vi "Actor Core.vi"(8 "error in":errorcluster, 11 "MLTFNC in":refnum<class "MLTFNC.lvclass">) -> (0 "error out":errorcluster, 3 "Actor out":refnum<class "Actor.lvclass">)   [LabVIEW 2019, in "MLTFNC.lvlib" / "MLTFNC.lvclass"]
doc: "The instrument actor core is only here to distribute panel resolution settings to children classes."
uses:
  Library/MLTFNC.lvclass
  builds/Engine/Actor Framework.lvlibp/1abvi3w/vi.lib/ActorFramework/Actor/Actor.lvclass
  MLTFNC Messages/Toggle Channel Msg/Toggle Channel Msg.lvclass/Toggle Channel Msg.ctl
  builds/Engine/Actor Framework.lvlibp/1abvi3w/vi.lib/ActorFramework/Message Enqueuer/Enqueue.vi
  MLTFNC Messages/Clear All Msg/Clear All Msg.lvclass
  MLTFNC Messages/Toggle Channel Msg/Toggle Channel Msg.lvclass
  builds/Instruments/Instruments.lvlibp/Library/Instruments.lvclass
  C:/Users/Public/Documents/Development/builds/Instruments/Instruments.lvlibp/Library/Instruments.lvclass
panel:
  in  "Active Device":u16(ring)
  in  "Active Routes":i32(listbox)
  in  "Route Bank 2":bool
  in  "Bank 2":u16(ring)
  in  "Unroute_Selected":bool
  in  "Route Bank 1":bool
  in  "Bank 1":u16(ring)
  in  "Clear All":bool
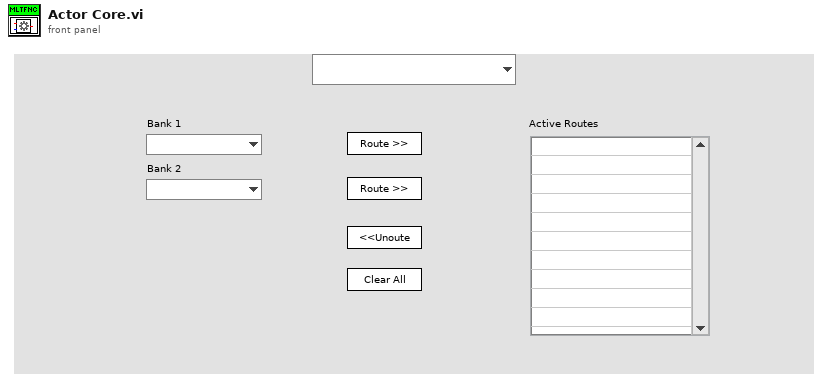
[diagram p1: front panel]
types:
  T1 = cluster{"Pnl Actor":refnum<event-registration>, "Event Registration Refnum":refnum<event-registration>}
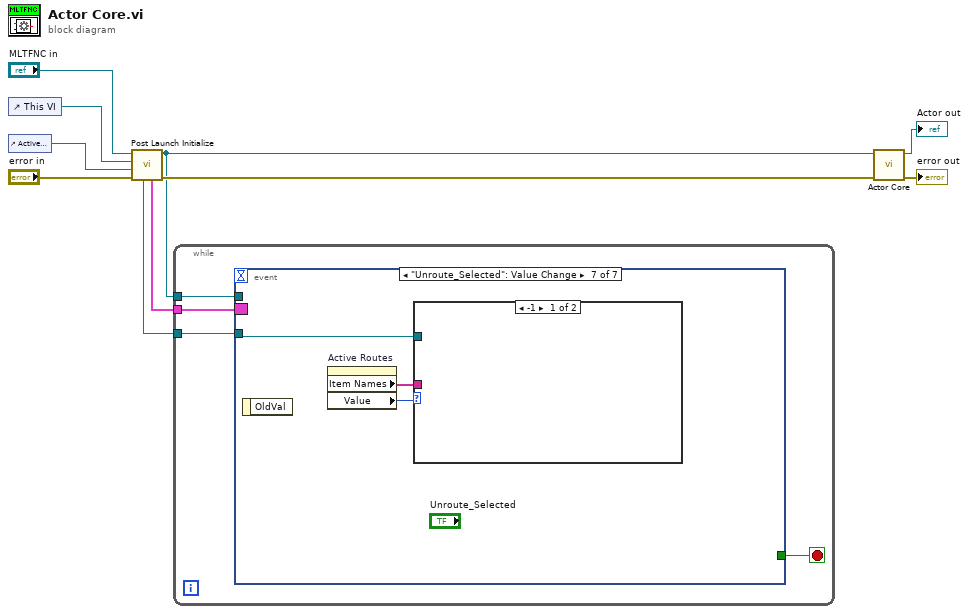
[diagram p0: block diagram]
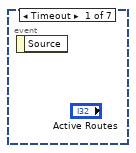
[diagram p2: hidden frame]
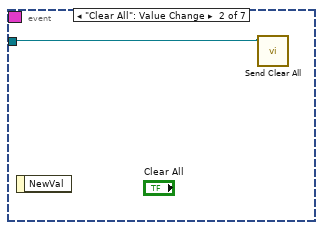
[diagram p3: hidden frame]
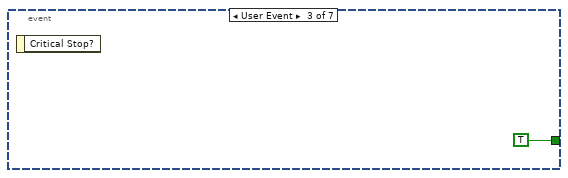
[diagram p4: hidden frame]
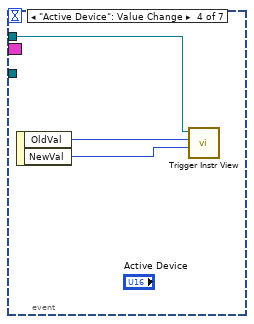
[diagram p5: hidden frame]
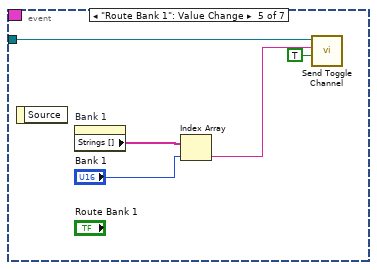
[diagram p6: hidden frame]
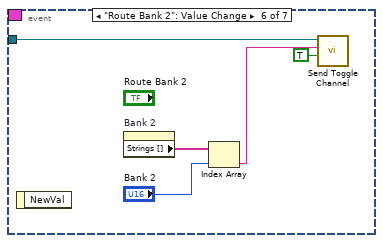
[diagram p7: hidden frame]
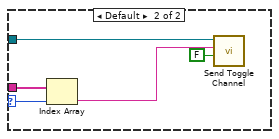
[diagram p8: hidden frame]
diagram:
  n1 = control-ref of="This VI"() -> (w2:refnum<vi>)
  n2 = control-ref of="Active Device"() -> (w3:refnum<vi>)
  n3 = call "Post Launch Initialize.vi"("error in"="error in", "Active Device"=w3, "GUI Reference"=w2, "Instruments in"="MLTFNC in") -> ("error out"=w6:errorcluster, "Instruments out"=w1:refnum<class "MLTFNC.lvclass">, "Registered Events"=w5:T1, "Self Enqueuer"=w4:refnum<class "Message Enqueuer.lvclass">)  [unwired: 4 in]
  n4 = while {
    tunnel: w5 -> [w14]
    tunnel: w4 -> [w11]
    tunnel: w1 -> [w13]
    stop <- w12 stop-if-true
    n5 = event shown="[6] \"Unroute_Selected\": Value Change" {
      selector: w14 -> [_ _ _ _ _ _ _]
      dyn-events: _ -> [_ _ _ _ _ _ _]
      timeout: _ -> [_ _ _ _ _ _ _]
      tunnel: w13 -> [_ _ _ w19 _ _ _]
      tunnel: [_ _ TRUE _ _ _ _] -> w12
      tunnel: w11 -> [_ w15 _ _ w24 w29 w31]
      event Timeout {
        n6 = event-data() -> ()  [unwired: 1 in, 1 out]
      }
      event "Clear All": Value Change {
        n7 = event-data() -> ()  [unwired: 1 in, 1 out]
        n8 = call "Send Clear All.vi"("Message Enqueuer"=w15) -> ()  [unwired: 9 in, 2 out]
      }
      event User Event {
        n9 = event-data() -> ()  [unwired: 1 in, 1 out]
      }
      event "Active Device": Value Change {
        n10 = event-data() -> ("OldVal"=w18:u16, "NewVal"=w17:u16)  [unwired: 1 in]
        n11 = call "Trigger Instr View.vi"("New Value"=w17, "Old Value"=w18, "Instruments in"=w19) -> ()  [unwired: 7 in, 2 out]
      }
      event "Route Bank 1": Value Change {
        n12 = event-data() -> ()  [unwired: 1 in, 1 out]
        n13 = property on="Bank 1" class="Ring (strict)"() -> ("Strings []"=w22:string[])  [unwired: 2 in, 2 out]
        n14 = Index Array(array=w22, index="Bank 1") -> (element=w20:string)
        n15 = call "Send Toggle Channel.vi"("State"=TRUE, "Name"=w20, "Message Enqueuer"=w24) -> ()  [unwired: 7 in, 2 out]
      }
      event "Route Bank 2": Value Change {
        n16 = event-data() -> ()  [unwired: 1 in, 1 out]
        n17 = property on="Bank 2" class="Ring (strict)"() -> ("Strings []"=w27:string[])  [unwired: 2 in, 2 out]
        n18 = Index Array(array=w27, index="Bank 2") -> (element=w25:string)
        n19 = call "Send Toggle Channel.vi"("State"=TRUE, "Name"=w25, "Message Enqueuer"=w29) -> ()  [unwired: 7 in, 2 out]
      }
      event "Unroute_Selected": Value Change {
        n20 = event-data() -> ()  [unwired: 1 in, 1 out]
        n21 = property on="Active Routes" class="LstBox (strict)"() -> ("Item Names"=w32:string[], "Value"=w30:i32)  [unwired: 2 in, 2 out]
        n22 = case shown="-1" w30 {
          selector: w30 -> [_ w33]
          tunnel: w32 -> [_ w37]
          tunnel: w31 -> [_ w36]
          frame -1 {
          }
          frame Default {
            n23 = Index Array(array=w37, index=w33) -> (element=w35:string)
            n24 = call "Send Toggle Channel.vi"("State"=FALSE, "Name"=w35, "Message Enqueuer"=w36) -> ()  [unwired: 7 in, 2 out]
          }
        }
      }
    }
  }
  n25 = call-parent "Actor Core.vi"("error in"=w6, "Instruments in"=w1) -> ("error out"=→"error out":errorcluster, "Actor out"=→"Actor out":refnum<class "Actor.lvclass">)  [unwired: 8 in]
